vi "Cannon Begin.vi"   [LabVIEW 2013]
uses:
  <vilib>/Rock Robotics/WPI/Solenoid/WPI_SolenoidChannel.ctl
  <vilib>/Rock Robotics/SystemInterfaces/Typedef/FPGA_TypedefSolenoidModule.ctl
  <vilib>/Rock Robotics/SystemInterfaces/DIO/FPGA_DIOChannel.ctl
  <vilib>/Rock Robotics/SystemInterfaces/Typedef/FPGA_TypedefAnalogModule.ctl
  <vilib>/Rock Robotics/SystemInterfaces/AI/FPGA_AIChannel.ctl
  <vilib>/Rock Robotics/SystemInterfaces/Typedef/FPGA_TypedefDigitalModule.ctl
  <vilib>/Rock Robotics/SystemInterfaces/DIO/FPGA_DIOPWMChannel.ctl
  <vilib>/Rock Robotics/WPI/Solenoid/WPI_SolenoidOpenDouble.vi
types:
  T1 = typedef "FPGA_DIOPWMChannel.ctl" = enum8{"PWM 1", "PWM 2", "PWM 3", "PWM 4", "PWM 5", "PWM 6", "PWM 7", "PWM 8", "PWM 9", "PWM 10", "Invalid"}
  T2 = typedef "FPGA_TypedefDigitalModule.ctl" = enum16{"Digital Module 1", "Digital Module 2"}
  T3 = typedef "FPGA_AIChannel.ctl" = enum8{"AI 1", "AI 2", "AI 3", "AI 4", "AI 5", "AI 6", "AI 7", "AI 8", "Invalid"}
  T4 = typedef "FPGA_TypedefAnalogModule.ctl" = enum16{"Analog Module 1", "Analog Module 2"}
  T5 = typedef "FPGA_DIOChannel.ctl" = enum8{"DIO 1", "DIO 2", "DIO 3", "DIO 4", "DIO 5", "DIO 6", "DIO 7", "DIO 8", "DIO 9", "DIO 10", "DIO 11", "DIO 12", "DIO 13", "DIO 14", "Invalid"}
  T6 = typedef "WPI_SolenoidChannel.ctl" = enum8{"Solenoid 1", "Solenoid 2", "Solenoid 3", "Solenoid 4", "Solenoid 5", "Solenoid 6", "Solenoid 7", "Solenoid 8", "Invalid"}
  T7 = typedef "FPGA_TypedefSolenoidModule.ctl" = enum16{"Solenoid Module 1", "Solenoid Module 2"}
  T8 = typedef "WPI_DigitalInputDevRef.ctl" = cluster{"DevStatus":errorcluster, "DIO Channel":T5, "Digital Module":T2}
  T9 = typedef "WPI_AnalogChannelDevRef.ctl" = cluster{"DevStatus":errorcluster, "Analog Module":T4, "Analog Channel":T3}
  T10 = typedef "WPI_SolenoidDevRef.ctl" = cluster{"DevStatus":errorcluster, "Solenoid Module":T7, "Forward Solenoid Channel":T6, "Reverse Solenoid Channel":T6}
  T11 = typedef "WPI_ServoDeviceRef.ctl" = cluster{"DeviceStatus":errorcluster, "Digital Module":T2, "PWM Channel":T1, "DeadBand":T12}
  T12 = typedef "WPI_PWMDeadband.ctl" = cluster{"Name":string, "maxPositivePwm":i32, "minPositivePwm":i32, "centerPwm":i32, "maxNegativePwm":i32, "minNegativePwm":i32, "angularRange":u16}
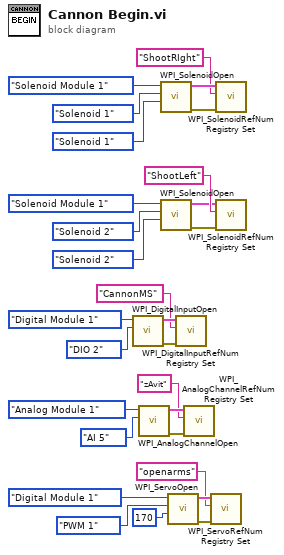
[diagram p0: block diagram]
diagram:
  n1 = call <vilib>:"WPI_DigitalInputOpen.vi"("DIO Channel"=FPGA_DIOChannel."DIO 2", "Digital Module (Module 1)"=FPGA_TypedefDigitalModule."Digital Module 1") -> ("error out"=w15:errorcluster, "DigitalInputDevRef"=w16:T8)  [unwired: 8 in]
  n2 = call <vilib>:"WPI_AnalogChannelOpen.vi"("Analog Channel"=FPGA_AIChannel."AI 5", "Analog Module (Module 1)"=FPGA_TypedefAnalogModule."Analog Module 1") -> ("error out"=w11:errorcluster, "AIDeviceRef"=w10:T9)  [unwired: 8 in]
  n3 = call-poly <vilib>:"WPI_SolenoidOpen.vi"("Reverse Solenoid Channel"=WPI_SolenoidChannel."Solenoid 1", "Forward Solenoid Channel"=WPI_SolenoidChannel."Solenoid 1", "Solenoid Module (Module 1)"=FPGA_TypedefSolenoidModule."Solenoid Module 1") -> ("error out"=w27:errorcluster, "SolenoidDevRef"=w28:T10)  [unwired: 7 in]
  n4 = call-poly <vilib>:"WPI_SolenoidOpen.vi"("Reverse Solenoid Channel"=WPI_SolenoidChannel."Solenoid 2", "Forward Solenoid Channel"=WPI_SolenoidChannel."Solenoid 2", "Solenoid Module (Module 1)"=FPGA_TypedefSolenoidModule."Solenoid Module 1") -> ("error out"=w18:errorcluster, "SolenoidDevRef"=w17:T10)  [unwired: 7 in]
  n5 = call <vilib>:"WPI_ServoOpen.vi"("Angular Range"=u16 170, "PWM Channel"=FPGA_DIOPWMChannel."PWM 1", "Digital Module (Module 1)"=FPGA_TypedefDigitalModule."Digital Module 1") -> ("error out"=w6:errorcluster, "ServoDeviceRef"=w5:T11)  [unwired: 7 in]
  n6 = call <vilib>:"WPI_DigitalInputRefNum Registry Set.vi"("error in (no error)"=w15, "refnum name"="CannonMS", "DigitalInputDevRef"=w16) -> ()  [unwired: 7 in, 2 out]
  n7 = call <vilib>:"WPI_AnalogChannelRefNum Registry Set.vi"("error in (no error)"=w11, "refnum name"="zAvit", "AIDeviceRef"=w10) -> ()  [unwired: 7 in, 2 out]
  n8 = call <vilib>:"WPI_ServoRefNum Registry Set.vi"("error in (no error)"=w6, "refnum name"="openarms", "ServoDeviceRef"=w5) -> ()  [unwired: 7 in, 2 out]
  n9 = call <vilib>:"WPI_SolenoidRefNum Registry Set.vi"("error in (no error)"=w27, "refnum name"="ShootRIght", "SolenoidDevRef"=w28) -> ()  [unwired: 7 in, 2 out]
  n10 = call <vilib>:"WPI_SolenoidRefNum Registry Set.vi"("error in (no error)"=w18, "refnum name"="ShootLeft", "SolenoidDevRef"=w17) -> ()  [unwired: 7 in, 2 out]
